vi "Diverse Einstellungen.vi"(8 "error in (no error)":errorcluster caption="Fehler (Eingang)") -> (0 "error out":errorcluster caption="Fehler (Ausgang)")   [LabVIEW 2020, in "FT-IR.lvlib"]
uses:
  FT-IR.lvlib
  FGV FT-IR Aktionen.ctl
  Funktionstasten/Funktionstasten-Aktion.ctl
  Funktionstasten/Zustaende.ctl
  Stoerungen/Stoerungen Messgeraet/Aktionen Kommunikation Stoerung.ctl
  Funktionstasten/Funktionstasten.lvlib
  TOOLweb Interface Library/TOOLweb Interface.lvlib
  Stoerungen/Stoerungen.lvlib
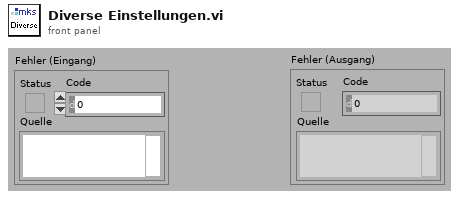
[diagram p1: front panel]
types:
  T1 = typedef "Stoerungen.lvlib/Aktionen Kommunikation Stoerung.ctl" = enum16{"lesen", "init", "FT-IR Komm", "FT-IR Betriebsart", "FT-IR Hintergrund", "cRIO Komm", "PNS Komm", "Dichtheitstest", "Life Bit", "FTIR Komm AK", "PMA Komm", "FID Komm", "PMA Cal", "FID Ch4 Cal", "FID THC Cal", "Cal Timeout", "VFS 1 Komm", "VFS 2 Komm", "VFS 3 Komm", "VFS 4 Komm", "TRE 08 Komm", "CG-Test vorzeitig", "CG-Test Span 1", "CG-Test Span 2", "CG-Test Span 3", "CG-Test Messgas", "CG-Test löschen", "Test", "Amium AK"}
  T2 = typedef "Funktionstasten.lvlib/Zustaende.ctl" = enum16{"Standby", "Pause", "Eco", "Messen", "Kalibrieren", "Spülen Filter", "Spülen Leitung", "Umgebungsluft", "0-Gas", "Cal-Gas", "CG zu PNS", "-------------", "Init 1", "Init 2", "Init 3", "Init 4", "Messen vorbereiten", "Messen durchführen", "Exit"}
  T3 = typedef "Funktionstasten.lvlib/Funktionstasten-Aktion.ctl" = enum16{"Initialisieren", "Zustand setzen", "Taste gedrückt", "Fehler speichern", "Lesen", "Manuell", "Remote", "Bitparallel", "Samplepoint", "Zeit Prüfen", "reset Umschalten"}
  T4 = typedef "FT-IR.lvlib/FGV FT-IR Aktionen.ctl" = enum16{"lesen", "NOG setzen", "NOS setzen", "Initialisieren", "speichern", "ALLES setzen", "FT-IR Spektrum loggen", "Komm Stoppen", "Spektrum LogKonfig"}
  T5 = typedef "FT-IR.lvlib/TOOLweb Interface.lvlib/Typdefinitionen.lvlib/TOOLweb Einstellungen.ctl" = cluster{"(1) InstrumentState":string, "(10) NrOfGasses":i32, "(21) recipeCurrent":string, "(80) labEnabled":bool, "(81) labPath":path, "(82) labBaseName":string, "(83) labIndex":string, "(90) ftirScans":i32}
  T6 = cluster{"(80) labEnabled":bool, "(81) labPath":path, "(82) labBaseName":string, "(83) labIndex":string, "Spektrum loggen aktiv?":bool}
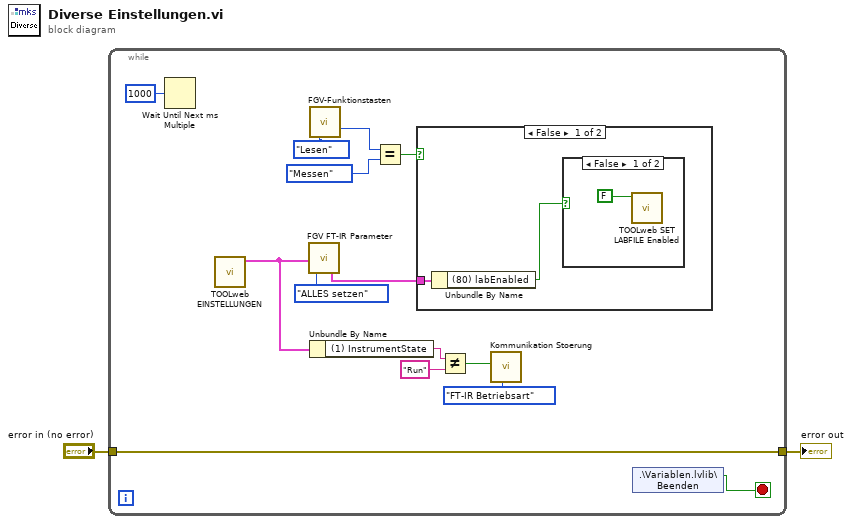
[diagram p0: block diagram]
diagram:
  n1 = while {
    tunnel: "error in (no error)" -> [w14]
    tunnel: [w14] -> w1
    stop <- w16 stop-if-true
    n2 = Wait Until Next ms Multiple(millisecond multiple=u32 1000 ("Vielfache von ms")) -> ()  [unwired: 1 out]
    n3 = call "TOOLweb EINSTELLUNGEN.vi"() -> ("Einstellungen"=w7:T5)  [unwired: 3 in, 4 out]
    n4 = call "FGV FT-IR Parameter.vi"("Einstellungen"=w7, "Aktion"=FGV_FT-IR_Aktionen."ALLES setzen") -> ("Ausgangs-Cluster"=w9:T6)  [unwired: 10 in, 7 out]
    n5 = call "FGV-Funktionstasten.vi"("Aktion"=Funktionstasten-Aktion."Lesen") -> ("ausgewählte Funktion"=w11:T2)  [unwired: 9 in, 5 out]
    n6 = Unbundle By Name(w7) -> ("(1) InstrumentState"=w5:string)
    n7 = Equal?(x=w11, y=Zustaende."Messen" ("ausgewählte Funktion")) -> (x = y?=w13:bool)
    n8 = case shown="False" w13 {
      tunnel: w9 -> [w18 _]
      frame False {
        n9 = Unbundle By Name(w18) -> ("(80) labEnabled"=w17:bool)
        n10 = case shown="False" w17 {
          frame False {
            n11 = call "TOOLweb SET LABFILE Enabled.vi"("Enabled"=FALSE) -> ()  [unwired: 2 in, 5 out]
          }
          frame True {
          }
        }
      }
      frame True {
      }
    }
    n12 = Not Equal?(x=w5, y="Run") -> (x != y?=w6:bool)
    n13 = call "Kommunikation Stoerung.vi"("Aktionen"=Aktionen_Kommunikation_Stoerung."FT-IR Betriebsart", "ERROR"=w6) -> ()  [unwired: 9 in, 1 out]
    n14 = shared-variable ".\\Variablen.lvlib\\Beenden"() -> (w16:bool)  [unwired: 1 in, 1 out]
  }
  "error out" <- w1
